vi "XML Read Value.vi"(6 "Default Attribute Values":variant[](array[variant]), 7 "Attribute Names":string[](array[string]), 8 "error in (no error)":errorcluster, 9 "Default Element Value":variant, 10 "Element Name":string, 11 "XML Reader In":T1) -> (0 "error out":errorcluster, 1 "Element Value":variant, 2 "Found?":bool, 3 "XML Reader Out":T1, 4 "Attribute Values":variant[](array[variant]))   [LabVIEW 2016, in "Pathloss XML Reader.lvlib"]
uses:
  Pathloss XML Reader.lvlib
  Controls/XML Reader Data Ref.ctl
  Controls/XML Reader Data.ctl
  <vilib>/Utility/VariantDataType/VariantType.lvlib
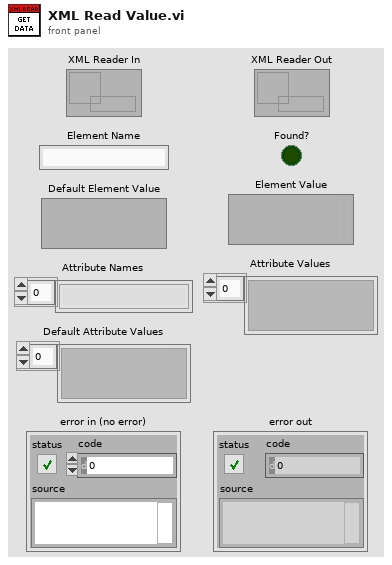
[diagram p1: front panel]
types:
  T1 = typedef "Pathloss XML Reader.lvlib/XML Reader Data Ref.ctl" = refnum<data-value>
  T2 = typedef "Pathloss XML Reader.lvlib/XML Reader Data.ctl" = cluster{"Remaining XML":string, "Section Name Stack":string[], "Section Stack":string[]}
  T3 = typedef "VariantType.lvlib/Type.ctl" = enum8{"Invalid Type", "Void", "I8", "I16", "I32", "I64", "U8", "U16", "U32", "U64", "Single Float", "Double Float", "Extended Float", "Single Complex", "Double Complex", "Extended Complex", "Enum U8", "Enum U16", "Enum U32", "Enum U64", "Single Float With Unit", "Double Float With Unit", "Extended Float With Unit", "Single Complex with Unit", "Double Complex with Unit", "Extended Complex with Unit", "Boolean", "String", "Path", "Picture", "Tag", "Array", "Cluster", "Variant", "LV Variant", "Waveform", "Timestamp", "Digital Waveform", "Digital Data", "ExpressData", "Refnum", "External Data", "VI", "Poly VI", "LabVIEW Class Instance", "Fixed Point"}
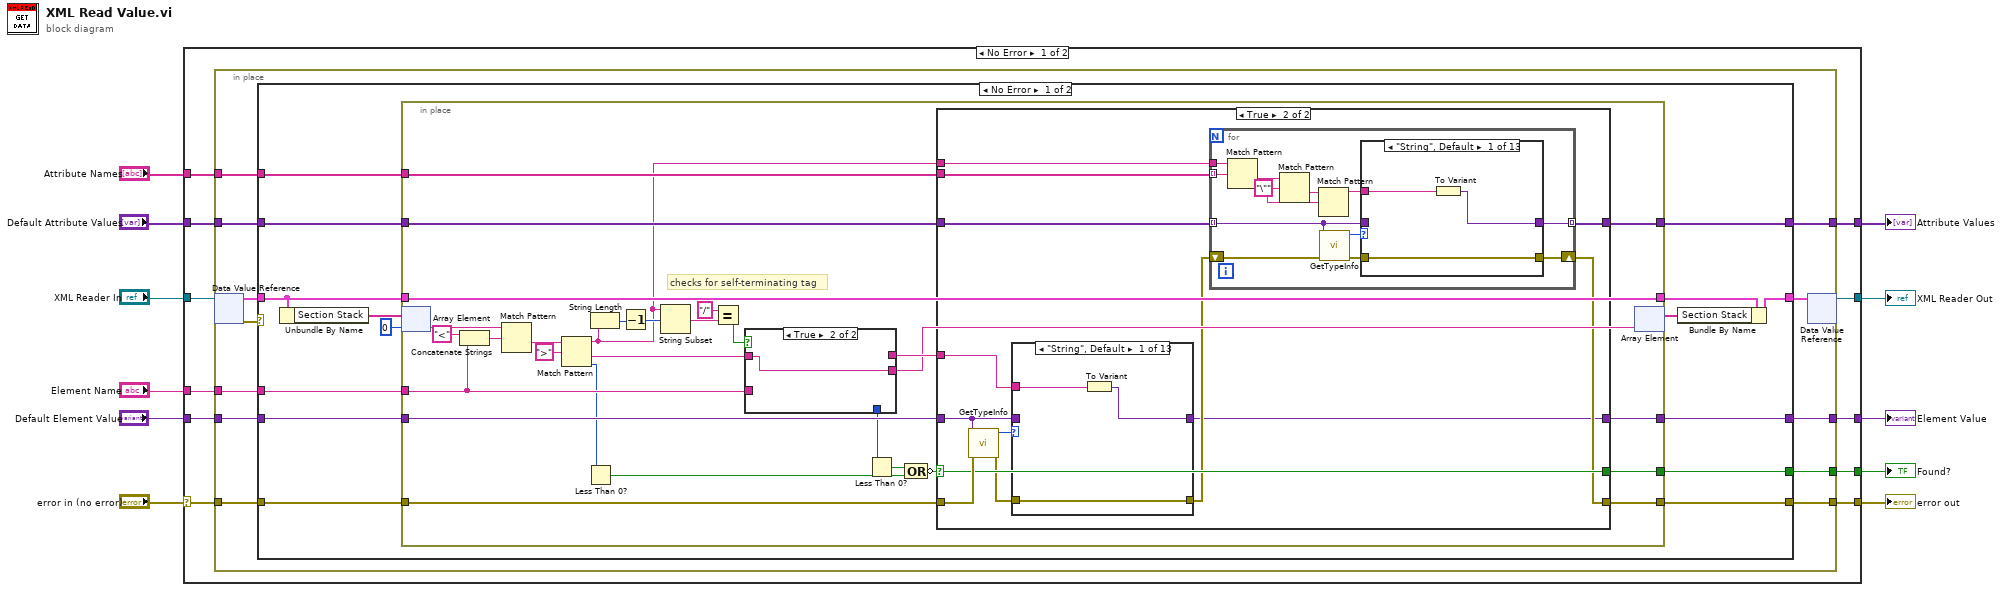
[diagram p0: block diagram]
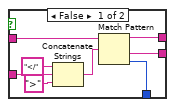
[diagram p2: hidden frame]
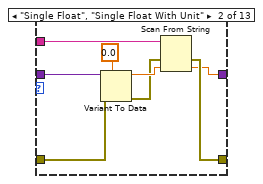
[diagram p4: hidden frame]
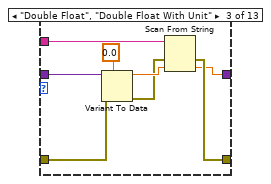
[diagram p5: hidden frame]
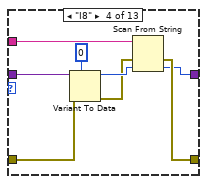
[diagram p6: hidden frame]
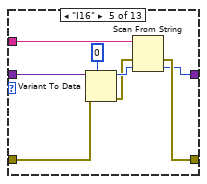
[diagram p7: hidden frame]
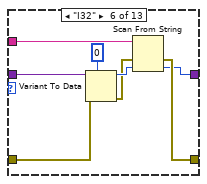
[diagram p8: hidden frame]
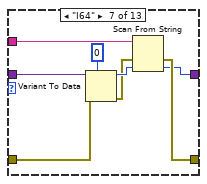
[diagram p9: hidden frame]
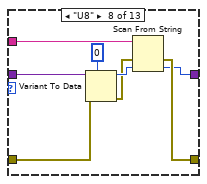
[diagram p10: hidden frame]
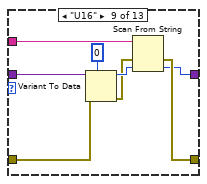
[diagram p11: hidden frame]
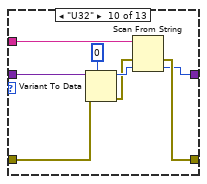
[diagram p12: hidden frame]
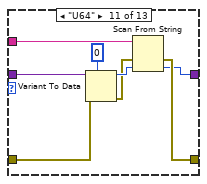
[diagram p13: hidden frame]
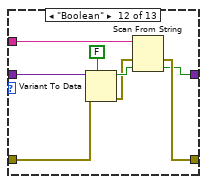
[diagram p14: hidden frame]
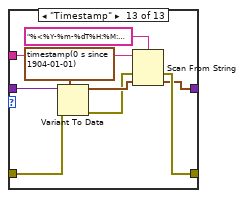
[diagram p15: hidden frame]
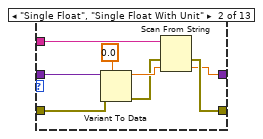
[diagram p16: hidden frame]
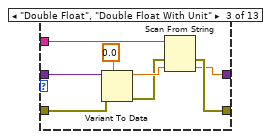
[diagram p17: hidden frame]
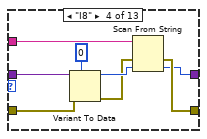
[diagram p18: hidden frame]
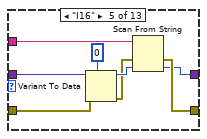
[diagram p19: hidden frame]
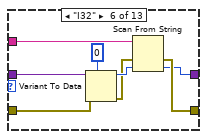
[diagram p20: hidden frame]
diagram:
  n1 = case shown="No Error" "error in (no error)" {
    selector: "error in (no error)" -> [w20 w323]
    tunnel: [w19 w323] -> w10
    tunnel: [w21 w324] -> w9
    tunnel: "XML Reader In" -> [w22 w324]
    tunnel: "Element Name" -> [w18 _]
    tunnel: "Attribute Names" -> [w17 _]
    tunnel: "Default Attribute Values" -> [w16 w322]
    tunnel: "Default Element Value" -> [w15 w321]
    tunnel: [w14 _] -> w1
    tunnel: [w13 w322] -> w4
    tunnel: [w12 w321] -> w2
    frame No Error {
      n2 = in-place {
        in-place-border: w20 -> [w31]
        in-place-border: [w30] -> w19
        in-place-border: w18 -> [w29]
        in-place-border: w17 -> [w28]
        in-place-border: w16 -> [w27]
        in-place-border: w15 -> [w26]
        in-place-border: [w25] -> w14
        in-place-border: [w24] -> w13
        in-place-border: [w23] -> w12
        n3 = in-place-dvr #1(w22) -> (w33:T2, w34:errorcluster)
        n4 = case shown="No Error" w34 {
          selector: w34 -> [_ w319]
          tunnel: w33 -> [w37 w320]
          tunnel: [w36 w320] -> w32
          tunnel: w31 -> [w49 _]
          tunnel: [w48 w319] -> w30
          tunnel: w29 -> [w46 _]
          tunnel: w28 -> [w42 _]
          tunnel: w27 -> [w43 w318]
          tunnel: w26 -> [w45 w317]
          tunnel: [w44 _] -> w25
          tunnel: [w41 w318] -> w24
          tunnel: [w40 w317] -> w23
          frame No Error {
            n5 = Unbundle By Name(w37) -> ("Section Stack"=w39:string[])
            n6 = in-place {
              in-place-border: w49 -> [w72]
              in-place-border: [w71] -> w48
              in-place-border: [w56] -> w47
              in-place-border: w46 -> [w68]
              in-place-border: w45 -> [w67]
              in-place-border: [w64] -> w44
              in-place-border: w43 -> [w63]
              in-place-border: w42 -> [w62]
              in-place-border: [w61] -> w41
              in-place-border: [w60] -> w40
              in-place-border: w37 -> [w56]
              # "checks for self-terminating tag"
              n7 = in-place-array #2(w39, 0) -> (w58:string)
              n8 = Concatenate Strings("<" ("string"), w68) -> (w77:string)
              n9 = Match Pattern(string=w58, regular expression=w77) -> (after substring=w76:string)  [unwired: 1 in, 3 out]
              n10 = Match Pattern(string=w76, regular expression=">") -> (before substring=w53:string, after substring=w70:string, offset past match=w65:i32)  [unwired: 1 in, 1 out]
              n11 = Less Than 0?(x=w65) -> (x < 0?=w74:bool)
              n12 = String Length(string=w53) -> (length=w55:i32)
              n13 = Decrement(x=w55) -> (x-1=w54:i32)
              n14 = String Subset(string=w53, offset (0)=w54) -> (substring=w52:string)  [unwired: 1 in]
              n15 = Equal?(x="/", y=w52) -> (x = y?=w50:bool)
              n16 = case shown="True" w50 {
                tunnel: w70 -> [w86 w87]
                tunnel: w68 -> [w83 _]
                tunnel: [w81 _] -> w66
                tunnel: [w80 _] -> w59
                tunnel: [w79 w87] -> w57
                frame False {
                  n17 = Concatenate Strings("</" ("string"), w83, ">" ("string")) -> (w82:string)
                  n18 = Match Pattern(string=w86, regular expression=w82) -> (before substring=w80:string, after substring=w79:string, offset past match=w81:i32)  [unwired: 1 in, 1 out]
                }
                frame True {
                }
              }
              n19 = Less Than 0?(x=w66) -> (x < 0?=w69:bool)
              n20 = Compound Arithmetic op=OR(w69, w74) -> (invert w73:bool)
              n21 = case shown="True" w73 {
                selector: w73 -> [w90 w103]
                tunnel: w72 -> [w91 w104]
                tunnel: [w91 w99] -> w71
                tunnel: w67 -> [w88 w93]
                tunnel: w53 -> [_ w101]
                tunnel: w59 -> [_ w97]
                tunnel: [w90 w103] -> w64
                tunnel: w63 -> [w89 w100]
                tunnel: w62 -> [_ w102]
                tunnel: [w89 w98] -> w61
                tunnel: [w88 w92] -> w60
                frame False {
                }
                frame True {
                  n22 = call <vilib>:"GetTypeInfo.vi"("error in (no error)"=w104, "Variant"=w93) -> ("error out"=w95:errorcluster, "Type Enum"=w96:T3)  [unwired: 5 in, 3 out]
                  n23 = case shown="\"String\", Default" w96 {
                    tunnel: w97 -> [w106 w115 w123 w131 w139 w147 w155 w163 w171 w179 w187 w195 w204]
                    tunnel: w93 -> [_ w114 w122 w130 w138 w146 w154 w162 w170 w178 w186 w194 w203]
                    tunnel: w95 -> [w107 w113 w121 w129 w137 w145 w153 w161 w169 w177 w185 w193 w202]
                    tunnel: [w107 w110 w118 w126 w134 w142 w150 w158 w166 w174 w182 w190 w199] -> w94
                    tunnel: [w105 w108 w116 w124 w132 w140 w148 w156 w164 w172 w180 w188 w197] -> w92
                    frame "String", Default {
                      n24 = To Variant(anything=w106) -> (Variant=w105:variant)
                    }
                    frame "Single Float", "Single Float With Unit" {
                      n25 = Variant To Data(error in=w113, type=sgl 0.0, Variant=w114) -> (data=w112:sgl, error out=w111:errorcluster)
                      n26 = Scan From String(input string=w115, error in=w111, default 1=w112) -> (error out=w110:errorcluster, output 1=w108:sgl)  [unwired: 2 in, 2 out]
                    }
                    frame "Double Float", "Double Float With Unit" {
                      n27 = Variant To Data(error in=w121, type=0.0, Variant=w122) -> (data=w120:dbl, error out=w119:errorcluster)
                      n28 = Scan From String(input string=w123, error in=w119, default 1=w120) -> (error out=w118:errorcluster, output 1=w116:dbl)  [unwired: 2 in, 2 out]
                    }
                    frame "I8" {
                      n29 = Variant To Data(error in=w129, type=i8 0, Variant=w130) -> (data=w128:i8, error out=w127:errorcluster)
                      n30 = Scan From String(input string=w131, error in=w127, default 1=w128) -> (error out=w126:errorcluster, output 1=w124:i8)  [unwired: 2 in, 2 out]
                    }
                    frame "I16" {
                      n31 = Variant To Data(error in=w137, type=i16 0, Variant=w138) -> (data=w136:i16, error out=w135:errorcluster)
                      n32 = Scan From String(input string=w139, error in=w135, default 1=w136) -> (error out=w134:errorcluster, output 1=w132:i16)  [unwired: 2 in, 2 out]
                    }
                    frame "I32" {
                      n33 = Variant To Data(error in=w145, type=0, Variant=w146) -> (data=w144:i32, error out=w143:errorcluster)
                      n34 = Scan From String(input string=w147, error in=w143, default 1=w144) -> (error out=w142:errorcluster, output 1=w140:i32)  [unwired: 2 in, 2 out]
                    }
                    frame "I64" {
                      n35 = Variant To Data(error in=w153, type=i64 0, Variant=w154) -> (data=w152:i64, error out=w151:errorcluster)
                      n36 = Scan From String(input string=w155, error in=w151, default 1=w152) -> (error out=w150:errorcluster, output 1=w148:i64)  [unwired: 2 in, 2 out]
                    }
                    frame "U8" {
                      n37 = Variant To Data(error in=w161, type=u8 0, Variant=w162) -> (data=w160:u8, error out=w159:errorcluster)
                      n38 = Scan From String(input string=w163, error in=w159, default 1=w160) -> (error out=w158:errorcluster, output 1=w156:u8)  [unwired: 2 in, 2 out]
                    }
                    frame "U16" {
                      n39 = Variant To Data(error in=w169, type=u16 0, Variant=w170) -> (data=w168:u16, error out=w167:errorcluster)
                      n40 = Scan From String(input string=w171, error in=w167, default 1=w168) -> (error out=w166:errorcluster, output 1=w164:u16)  [unwired: 2 in, 2 out]
                    }
                    frame "U32" {
                      n41 = Variant To Data(error in=w177, type=u32 0, Variant=w178) -> (data=w176:u32, error out=w175:errorcluster)
                      n42 = Scan From String(input string=w179, error in=w175, default 1=w176) -> (error out=w174:errorcluster, output 1=w172:u32)  [unwired: 2 in, 2 out]
                    }
                    frame "U64" {
                      n43 = Variant To Data(error in=w185, type=u64 0, Variant=w186) -> (data=w184:u64, error out=w183:errorcluster)
                      n44 = Scan From String(input string=w187, error in=w183, default 1=w184) -> (error out=w182:errorcluster, output 1=w180:u64)  [unwired: 2 in, 2 out]
                    }
                    frame "Boolean" {
                      n45 = Variant To Data(error in=w193, type=FALSE, Variant=w194) -> (data=w192:bool, error out=w191:errorcluster)
                      n46 = Scan From String(input string=w195, error in=w191, default 1=w192) -> (error out=w190:errorcluster, output 1=w188:bool)  [unwired: 2 in, 2 out]
                    }
                    frame "Timestamp" {
                      n47 = Variant To Data(error in=w202, type=timestamp(0 s since 1904-01-01), Variant=w203) -> (data=w201:timestamp, error out=w200:errorcluster)
                      n48 = Scan From String(format string="%<%Y-%m-%dT%H:%M:%S%7u%z>T" ("regular expression"), input string=w204, error in=w200, default 1=w201) -> (error out=w199:errorcluster, output 1=w197:timestamp)  [unwired: 1 in, 2 out]
                    }
                  }
                  n49 = for {
                    tunnel: w101 -> [w216]
                    tunnel: w102 -> [w215] mode=indexing
                    tunnel: w100 -> [w208] mode=indexing
                    shift-right: [w206] -> w99
                    shift-left: w94 -> [w211]
                    tunnel: [w205] -> w98 mode=indexing
                    w212 = "\"" ("regular expression")
                    n50 = Match Pattern(string=w216, regular expression=w215) -> (after substring=w214:string)  [unwired: 1 in, 3 out]
                    n51 = Match Pattern(string=w214, regular expression=w212) -> (after substring=w213:string)  [unwired: 1 in, 3 out]
                    n52 = Match Pattern(string=w213, regular expression=w212) -> (before substring=w209:string)  [unwired: 1 in, 3 out]
                    n53 = call <vilib>:"GetTypeInfo.vi"("error in (no error)"=w211, "Variant"=w208) -> ("error out"=w207:errorcluster, "Type Enum"=w210:T3)  [unwired: 5 in, 3 out]
                    n54 = case shown="\"String\", Default" w210 {
                      tunnel: w209 -> [w218 w227 w235 w243 w251 w259 w267 w275 w283 w291 w299 w307 w316]
                      tunnel: w208 -> [_ w226 w234 w242 w250 w258 w266 w274 w282 w290 w298 w306 w315]
                      tunnel: w207 -> [w219 w225 w233 w241 w249 w257 w265 w273 w281 w289 w297 w305 w314]
                      tunnel: [w219 w222 w230 w238 w246 w254 w262 w270 w278 w286 w294 w302 w311] -> w206
                      tunnel: [w217 w220 w228 w236 w244 w252 w260 w268 w276 w284 w292 w300 w309] -> w205
                      frame "String", Default {
                        n55 = To Variant(anything=w218) -> (Variant=w217:variant)
                      }
                      frame "Single Float", "Single Float With Unit" {
                        n56 = Variant To Data(error in=w225, type=sgl 0.0, Variant=w226) -> (data=w224:sgl, error out=w223:errorcluster)
                        n57 = Scan From String(input string=w227, error in=w223, default 1=w224) -> (error out=w222:errorcluster, output 1=w220:sgl)  [unwired: 2 in, 2 out]
                      }
                      frame "Double Float", "Double Float With Unit" {
                        n58 = Variant To Data(error in=w233, type=0.0, Variant=w234) -> (data=w232:dbl, error out=w231:errorcluster)
                        n59 = Scan From String(input string=w235, error in=w231, default 1=w232) -> (error out=w230:errorcluster, output 1=w228:dbl)  [unwired: 2 in, 2 out]
                      }
                      frame "I8" {
                        n60 = Variant To Data(error in=w241, type=i8 0, Variant=w242) -> (data=w240:i8, error out=w239:errorcluster)
                        n61 = Scan From String(input string=w243, error in=w239, default 1=w240) -> (error out=w238:errorcluster, output 1=w236:i8)  [unwired: 2 in, 2 out]
                      }
                      frame "I16" {
                        n62 = Variant To Data(error in=w249, type=i16 0, Variant=w250) -> (data=w248:i16, error out=w247:errorcluster)
                        n63 = Scan From String(input string=w251, error in=w247, default 1=w248) -> (error out=w246:errorcluster, output 1=w244:i16)  [unwired: 2 in, 2 out]
                      }
                      frame "I32" {
                        n64 = Variant To Data(error in=w257, type=0, Variant=w258) -> (data=w256:i32, error out=w255:errorcluster)
                        n65 = Scan From String(input string=w259, error in=w255, default 1=w256) -> (error out=w254:errorcluster, output 1=w252:i32)  [unwired: 2 in, 2 out]
                      }
                      frame "I64" {
                        n66 = Variant To Data(error in=w265, type=i64 0, Variant=w266) -> (data=w264:i64, error out=w263:errorcluster)
                        n67 = Scan From String(input string=w267, error in=w263, default 1=w264) -> (error out=w262:errorcluster, output 1=w260:i64)  [unwired: 2 in, 2 out]
                      }
                      frame "U8" {
                        n68 = Variant To Data(error in=w273, type=u8 0, Variant=w274) -> (data=w272:u8, error out=w271:errorcluster)
                        n69 = Scan From String(input string=w275, error in=w271, default 1=w272) -> (error out=w270:errorcluster, output 1=w268:u8)  [unwired: 2 in, 2 out]
                      }
                      frame "U16" {
                        n70 = Variant To Data(error in=w281, type=u16 0, Variant=w282) -> (data=w280:u16, error out=w279:errorcluster)
                        n71 = Scan From String(input string=w283, error in=w279, default 1=w280) -> (error out=w278:errorcluster, output 1=w276:u16)  [unwired: 2 in, 2 out]
                      }
                      frame "U32" {
                        n72 = Variant To Data(error in=w289, type=u32 0, Variant=w290) -> (data=w288:u32, error out=w287:errorcluster)
                        n73 = Scan From String(input string=w291, error in=w287, default 1=w288) -> (error out=w286:errorcluster, output 1=w284:u32)  [unwired: 2 in, 2 out]
                      }
                      frame "U64" {
                        n74 = Variant To Data(error in=w297, type=u64 0, Variant=w298) -> (data=w296:u64, error out=w295:errorcluster)
                        n75 = Scan From String(input string=w299, error in=w295, default 1=w296) -> (error out=w294:errorcluster, output 1=w292:u64)  [unwired: 2 in, 2 out]
                      }
                      frame "Boolean" {
                        n76 = Variant To Data(error in=w305, type=FALSE, Variant=w306) -> (data=w304:bool, error out=w303:errorcluster)
                        n77 = Scan From String(input string=w307, error in=w303, default 1=w304) -> (error out=w302:errorcluster, output 1=w300:bool)  [unwired: 2 in, 2 out]
                      }
                      frame "Timestamp" {
                        n78 = Variant To Data(error in=w314, type=timestamp(0 s since 1904-01-01), Variant=w315) -> (data=w313:timestamp, error out=w312:errorcluster)
                        n79 = Scan From String(format string="%<%Y-%m-%dT%H:%M:%S%7u%z>T" ("regular expression"), input string=w316, error in=w312, default 1=w313) -> (error out=w311:errorcluster, output 1=w309:timestamp)  [unwired: 1 in, 2 out]
                      }
                    }
                  }
                }
              }
              n80 = in-place-array #2(w57) -> (w35:string[])  [unwired: 1 out]
            }
            n81 = Bundle By Name(cluster=w47, "Section Stack"=w35) -> (w36:T2)
          }
          frame Error {
          }
        }
        n82 = in-place-dvr #1(w32) -> (w21:T1)  [unwired: 1 out]
      }
    }
    frame Error {
    }
  }
  "error out" <- w10
  "XML Reader Out" <- w9
  "Element Value" <- w2
  "Attribute Values" <- w4
  "Found?" <- w1
